vi "Get Lines.vi"() -> ()   [LabVIEW 2012]
uses:
  <vilib>/vision/Image Controls.llb/IMAQ Image.ctl
panel:
  out "XY Graph":cluster{dbl[], dbl[]}(graph)
  out "Lines Calibrated (Shape Detection 1)":T1(array[cluster]) {"End Point"."Y" format="%.2f"; "End Point"."X" format="%.2f"; "Start Point"."Y" format="%.2f"; "Start Point"."X" format="%.2f"}
  out "Image Out":T2
  in  "Image Name":string="untitled"
  in  "error in":errorcluster
  in  "Start Path":path
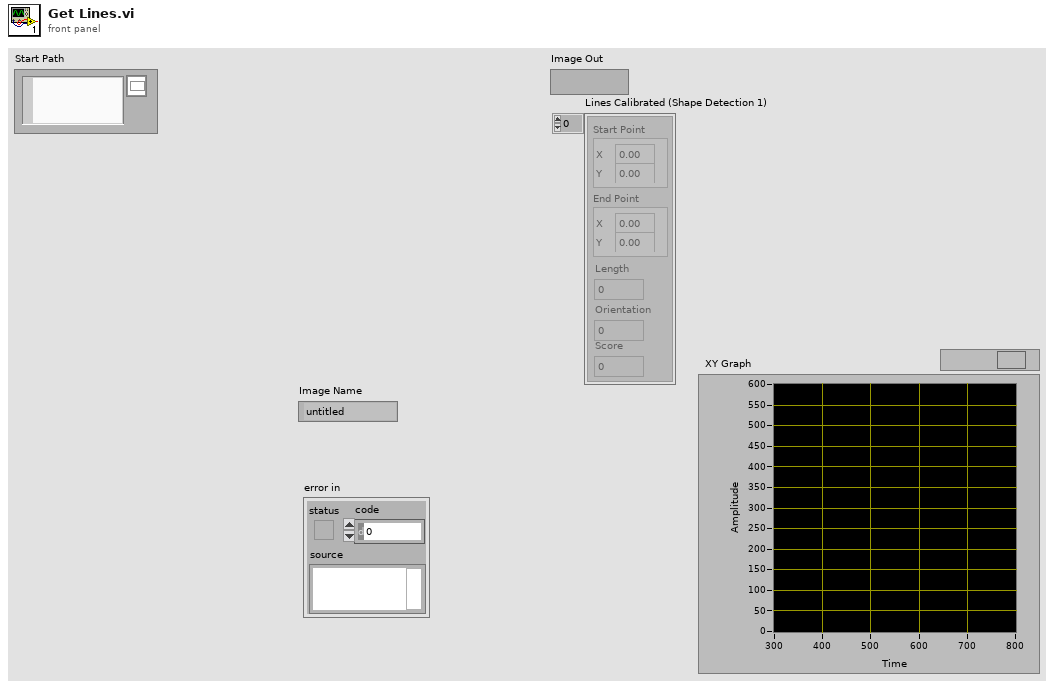
[diagram p1: front panel]
types:
  T1 = cluster{"Start Point":cluster{"X":sgl, "Y":sgl}, "End Point":cluster{"X":sgl, "Y":sgl}, "Length":dbl, "Orientation":dbl, "Score":dbl}[]
  T2 = typedef "IMAQ Image.ctl" = refnum<image>
  T3 = typedef "Image Type" = u32
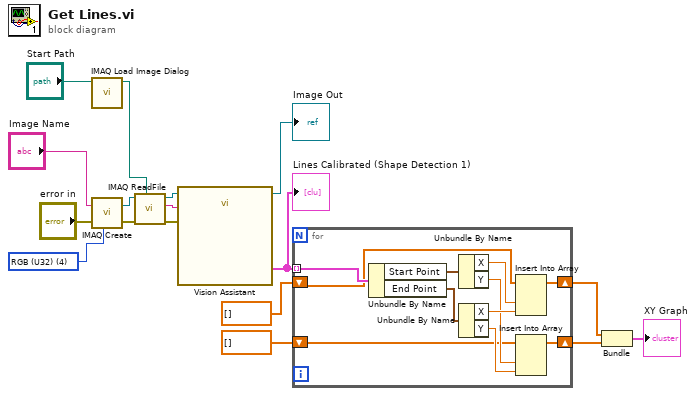
[diagram p0: block diagram]
diagram:
  w13 = T3 4 items=["Grayscale (U8)", "Grayscale (I16)", "Grayscale (SGL)", "Complex (CSG)", "RGB (U32)", "HSL (U32)", "RGB (U64)", "Grayscale (U16)"] ("Image Type")
  n1 = call "IMAQ Load Image Dialog"("Start Path"="Start Path") -> ("Path"=w16:path)  [unwired: 8 in, 2 out]
  n2 = call "IMAQ Create"("Image Name"="Image Name", "Image Type"=w13, "error in (no error)"="error in") -> ("New Image"=w12:T2, "error out"=w8:errorcluster)  [unwired: 2 in]
  n3 = call "IMAQ ReadFile"("File Path"=w16, "error in (no error)"=w8, "Image"=w12) -> ("error out"=w11:errorcluster, "File Type out"=w10:string, "Image Out"=w9:T2)  [unwired: 4 in, 2 out]
  n4 = call "Vision Assistant"("Image In"=w9, "Image Dst"=w10, "error in"=w11) -> ("Image Out"=→"Image Out":T2, "Lines Calibrated (Shape Detection 1)"=w1:T1)  [unwired: 21 in, 2 out]
  "Lines Calibrated (Shape Detection 1)" <- w1
  n5 = for {
    tunnel: w1 -> [w28] mode=indexing
    shift-right: [w20] -> w3
    shift-left: dbl[] [] -> [w27]
    shift-right: [w18] -> w2
    shift-left: dbl[] [] -> [w19]
    n6 = Unbundle By Name(w28) -> ("Start Point"=w25:cluster{"X":sgl, "Y":sgl}, "End Point"=w26:cluster{"X":sgl, "Y":sgl})
    n7 = Unbundle By Name(w25) -> ("X"=w24:sgl, "Y"=w22:sgl)
    n8 = Unbundle By Name(w26) -> ("X"=w23:sgl, "Y"=w21:sgl)
    n9 = Insert Into Array(array=w27, new element #1=w24, new element #2=w23) -> (w20:dbl[])  [unwired: 1 in]
    n10 = Insert Into Array(array=w19, new element #1=w22, new element #2=w21) -> (w18:dbl[])  [unwired: 1 in]
  }
  n11 = Bundle(w3, w2) -> (→"XY Graph":cluster{dbl[], dbl[]})  [unwired: 1 in]
